vi "Write Analogue.vi"(8 "error in (no error)":errorcluster, 9 "output":bool, 10 "Channel index":i32, 11 "HiPOT Instrument":refnum<class "HiPOT Instrument.lvclass">) -> (0 "error out":errorcluster, 2 "Success?":bool=TRUE, 3 "HiPOT Instrument out":refnum<class "HiPOT Instrument.lvclass">)   [LabVIEW 2025, in "HiPOT.lvlib" / "HiPOT Instrument.lvclass"]
uses:
  HiPOT Instrument.lvclass
  HiPOT Instrument.lvclass/HiPOT Instrument.ctl
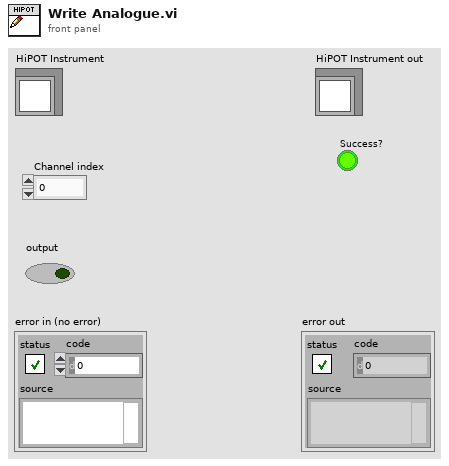
[diagram p1: front panel]
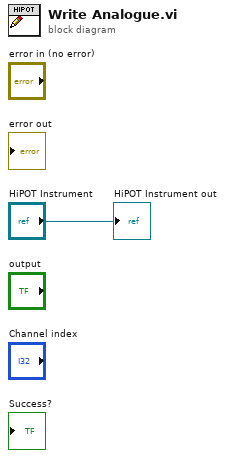
[diagram p0: block diagram]
diagram:
  "HiPOT Instrument out" <- "HiPOT Instrument"
